vi "Square.vi"   [LabVIEW 2016, in "xy_utilities.lvlib"]
doc: "Square <b>XY-data</b>'s y array.\n\nWire data to the data input to determine the polymorphic instance to use or manually select the instance."
uses:
  xy_utilities.lvlib
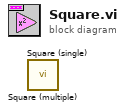
[diagram p0: block diagram]
diagram:
  n1 = call "Square (multiple).vi"() -> ()  [unwired: 10 in, 2 out]
  n2 = call "Square (single).vi"() -> ()  [unwired: 10 in, 2 out]
